vi "Parte2.vi"() -> ()   [LabVIEW 2016]
uses:
  <vilib>/Instr/_visa.llb/VISA Configure Serial Port (Instr).vi
panel:
  out "string":string
  out "Array 2":bool[](array[boolean])
  in  "Array":bool[](array[boolean])
  in  "Stop Button":bool
  in  "Cluster":T1={"VISA resource name"="", "baud rate (9600)"=9600, "data bits (8)"=8, "error in (no error)"={"status"=FALSE, "code"=0, "source"=""}, "parity (0:none)"=0, "stop bits (10: 1 bit)"=10, "flow control (0:none)"=0} {"flow control (0:none)" items=["None", "XON/XOFF", "RTS/CTS", "XON/XOFF & RTS/CTS", "DTR/DSR", "XON/XOFF & DTR/DSR"]; "stop bits (10: 1 bit)" items=["1.0"=10, "1.5"=15, "2.0"=20]; "parity (0:none)" items=["None", "Odd", "Even", "Mark", "Space"]; "data bits (8)" min=5 max=8 step=1}
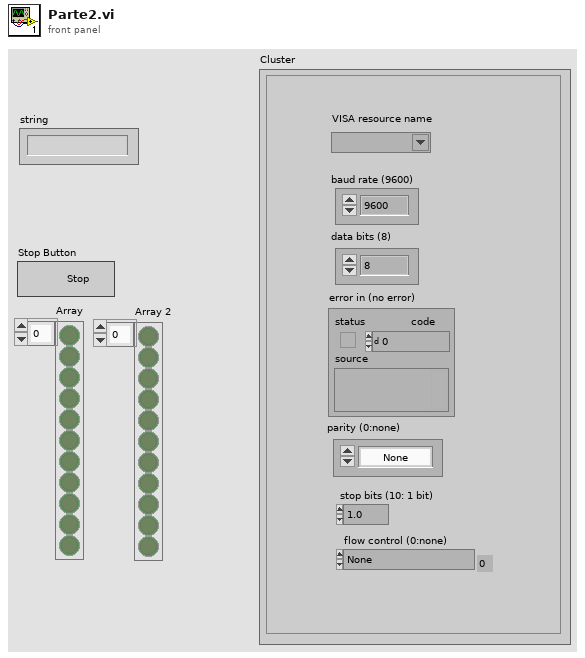
[diagram p1: front panel]
types:
  T1 = cluster{"VISA resource name":refnum<visa-resource-name>, "baud rate (9600)":u32, "data bits (8)":u16, "error in (no error)":errorcluster, "parity (0:none)":u16, "stop bits (10: 1 bit)":u16, "flow control (0:none)":u16}
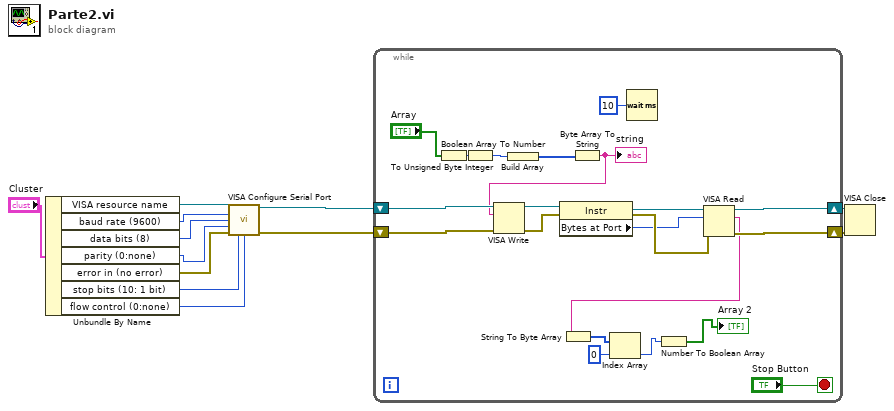
[diagram p0: block diagram]
diagram:
  n1 = Unbundle By Name("Cluster") -> ("VISA resource name"=w7:refnum<visa-resource-name>, "baud rate (9600)"=w8:u32, "data bits (8)"=w9:u16, "parity (0:none)"=w10:u16, "error in (no error)"=w11:errorcluster, "stop bits (10: 1 bit)"=w4:u16, "flow control (0:none)"=w3:u16)
  n2 = call-poly "VISA Configure Serial Port"("VISA resource name"=w7, "baud rate (9600)"=w8, "data bits (8)"=w9, "parity (0:none)"=w10, "error in (no error)"=w11, "stop bits (10: 1 bit)"=w4, "flow control (0:none)"=w3) -> ("VISA resource name out"=w6:refnum<visa-resource-name>, "error out"=w5:errorcluster)  [unwired: 7 in]
  n3 = while {
    shift-right: [w31] -> w2
    shift-left: w6 -> [w33]
    shift-right: [w30] -> w1
    shift-left: w5 -> [w32]
    stop <- "Stop Button" stop-if-true
    n4 = Boolean Array To Number(Boolean array="Array") -> (number=w22:u32)
    n5 = To Unsigned Byte Integer(number=w22) -> (unsigned 8bit integer=w21:u8)
    n6 = Build Array(w21) -> (w20:u8[])
    n7 = Byte Array To String(unsigned byte array=w20) -> (string=w18:string)
    "string" <- w18
    n8 = VISA Write(VISA resource name=w33, write buffer=w18, error in (no error)=w32) -> (VISA resource name out=w29:refnum<visa-resource-name>, error out=w28:errorcluster)  [unwired: 1 out]
    n9 = property class="Instr"(reference=w29, error in=w28) -> (reference out=w27:refnum<visa-resource-name>, error out=w26:errorcluster, "Bytes at Port"=w25:u32)
    n10 = Wait (ms)(milliseconds to wait=u32 10) -> ()  [unwired: 1 out]
    n11 = VISA Read(VISA resource name=w27, byte count=w25, error in (no error)=w26) -> (VISA resource name out=w31:refnum<visa-resource-name>, read buffer=w17:string, error out=w30:errorcluster)  [unwired: 1 out]
    n12 = String To Byte Array(string=w17) -> (unsigned byte array=w16:u8[])
    n13 = Index Array(array=w16, index=0) -> (element=w14:u8)
    n14 = Number To Boolean Array(number=w14) -> (Boolean array=→"Array 2":bool[])
  }
  n15 = VISA Close(VISA resource name=w2, error in (no error)=w1) -> ()  [unwired: 1 out]
